vi "Load Material Dialog.vi"(8 "error in":errorcluster, 9 "Material.Details":T2={"Font Name"="Segoe UI", "Button.Font Size"=30, "Message.Font Size"=30, "Message.Justification"=enum."Center", "Picture Background"=16777216}, 10 "Material.Scheme":T1) -> (0 "error out":errorcluster, 3 "Theme Obj":refnum<class "Theme.lvclass">)   [LabVIEW 2021, in "Theme.lvclass"]
doc: "Load a theme from a material file supported by the TSC Material Library:\n\nhttps://github.com/danielcoons/tsc-material-theme\nhttps://www.vipm.io/package/tsc_lib_tsc_material_theme/\n\n<b>Code Developed By:</b>\nTechnology Service Corporation\n1983 S Liberty Drive\nBloomington, IN 47403\nPhone: 812 558-7100\nwww.tsc.com/atcs\n\nDeveloper:\nDaniel Coons"
uses:
  Theme.lvclass
  Material.Details--typedef.ctl
  Material.Scheme--typedef.ctl
  Button colors--typedef.ctl
  message box--typdef.ctl
  Dialog colors--typedef.ctl
  Theme.lvclass/Theme.ctl
  Popup/PopUp Theme Global.vi
  Popup/Popup.lvclass
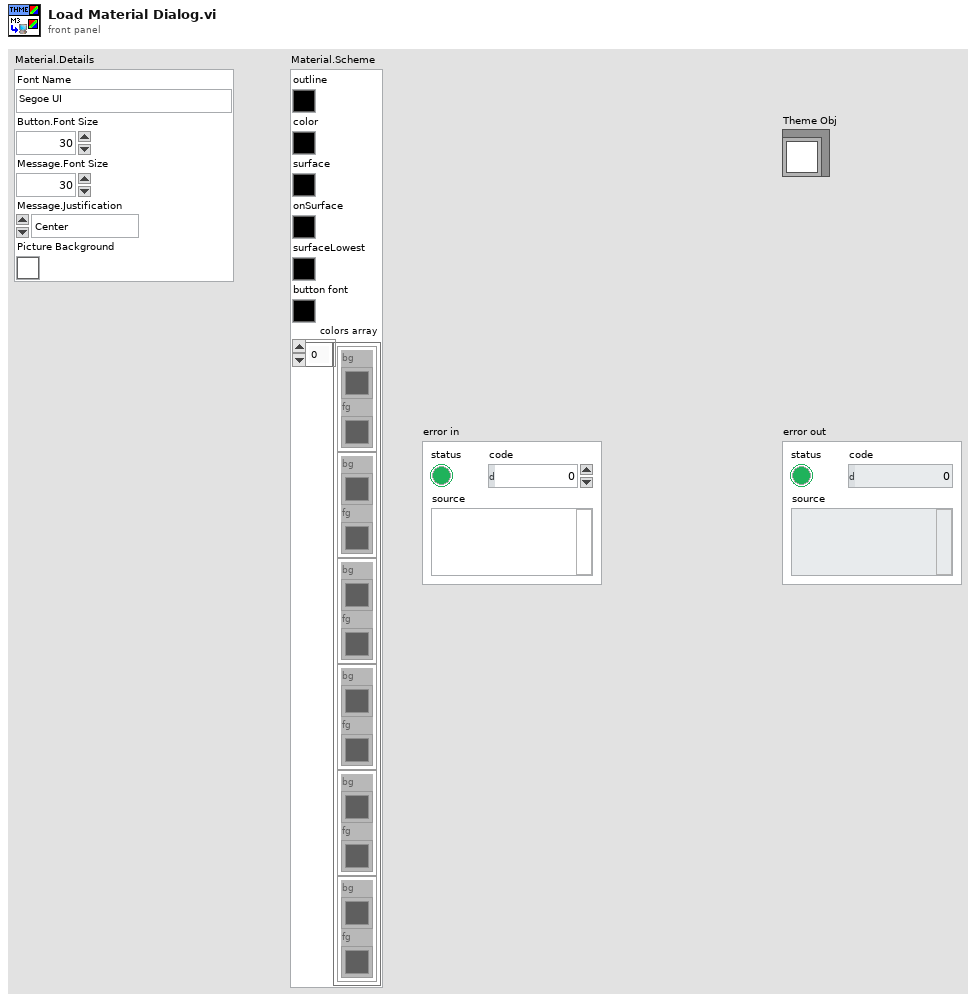
[diagram p1: front panel]
types:
  T1 = typedef "Theme.lvclass/Material.Scheme--typedef.ctl" = cluster{"outline":u32, "color":u32, "surface":u32, "onSurface":u32, "surfaceLowest":u32, "button font":u32, "colors array":cluster{"bg":u32, "fg":u32}[]}
  T2 = typedef "Theme.lvclass/Material.Details--typedef.ctl" = cluster{"Font Name":string, "Button.Font Size":u32, "Message.Font Size":u32, "Message.Justification":enum16{"Left", "Center", "Right"}, "Picture Background":u32}
  T3 = typedef "Theme.lvclass/Dialog colors--typedef.ctl" = cluster{"Header":u32, "Background":u32, "Picture Background":u32}
  T4 = typedef "Theme.lvclass/message box--typdef.ctl" = cluster{"Text.Font Name":string, "Text.Font Size":u32, "Color":u32, "Text.Justification":enum16{"Left", "Center", "Right"}, "messge color":cluster{"border":u32, "fill":u32}}
  T5 = typedef "Theme.lvclass/Button colors--typedef.ctl" = cluster{"false color":cluster{"border":u32, "fill":u32}, "hover color":cluster{"border":u32, "fill":u32}, "press color":cluster{"border":u32, "fill":u32}, "Boolean Text":u32, "Text.Font Name":string, "Text.Font Size":u32, "Bold?":bool, "Itallic?":bool}
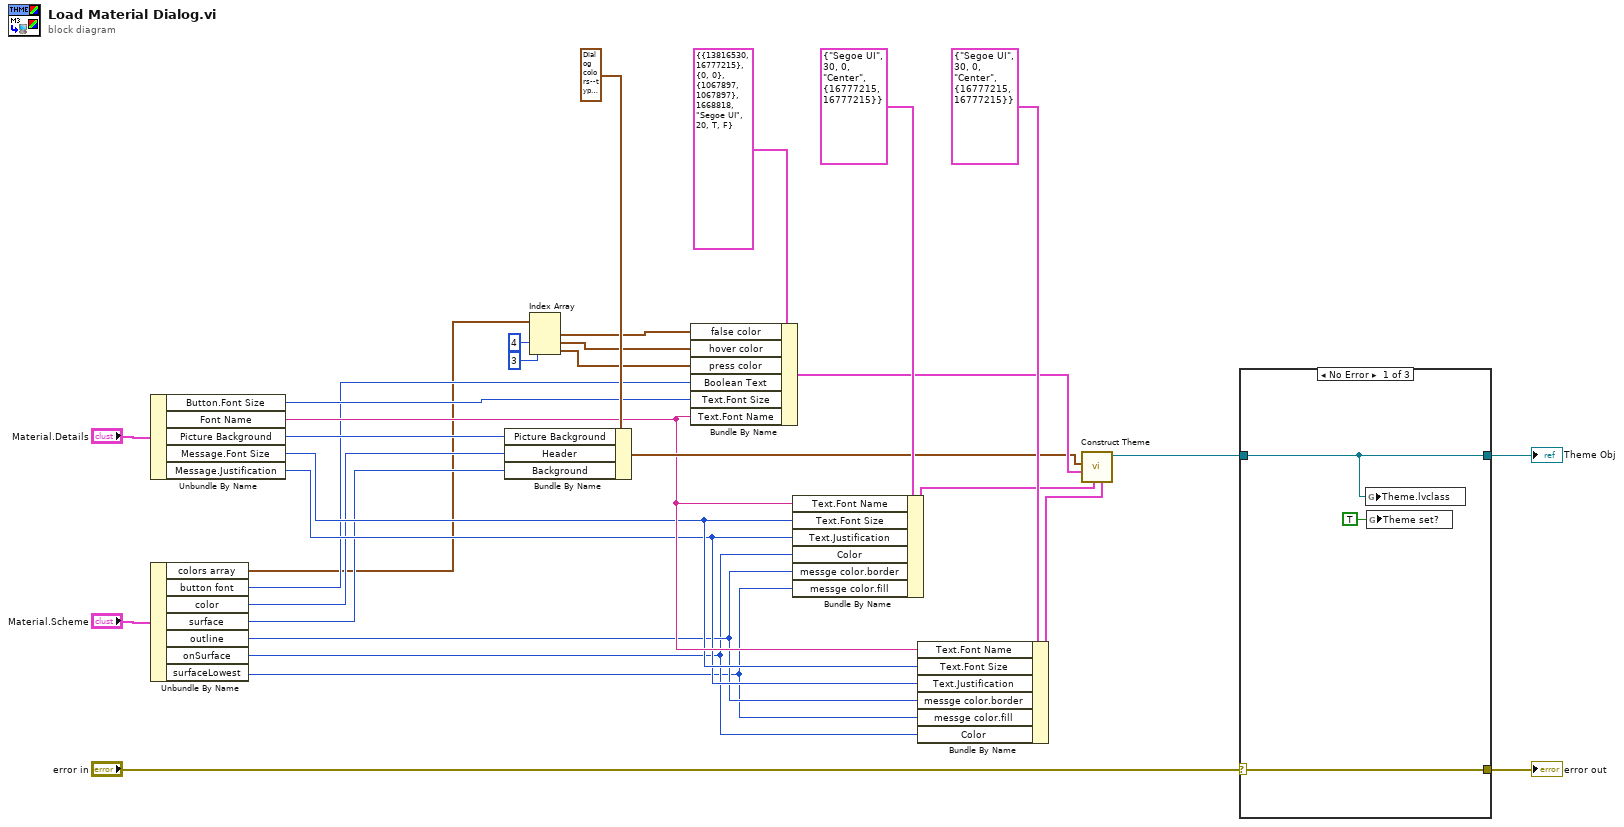
[diagram p0: block diagram]
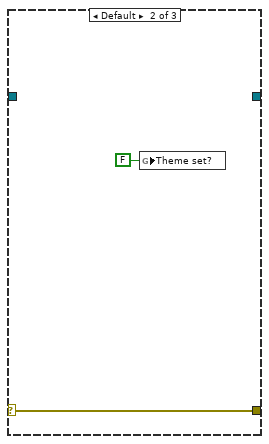
[diagram p2: hidden frame]
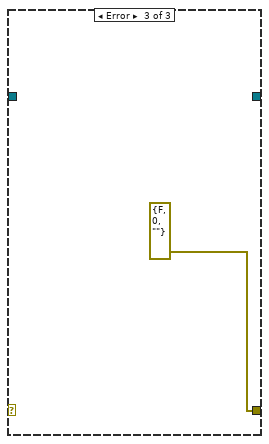
[diagram p3: hidden frame]
diagram:
  n1 = Unbundle By Name("Material.Details") -> ("Button.Font Size"=w13:u32, "Font Name"=w12:string, "Picture Background"=w11:u32, "Message.Font Size"=w10:u32, "Message.Justification"=w9:enum16{"Left", "Center", "Right"})
  n2 = Unbundle By Name("Material.Scheme") -> ("colors array"=w1:cluster{"bg":u32, "fg":u32}[], "button font"=w2:u32, "color"=w7:u32, "surface"=w5:u32, "outline"=w6:u32, "onSurface"=w4:u32, "surfaceLowest"=w3:u32)
  n3 = Bundle By Name(cluster=T3 {"Header"=1668818, "Background"=1668818, "Picture Background"=16777216} ("dialog colors"), "Picture Background"=w11, "Header"=w7, "Background"=w5) -> (w20:T3)
  n4 = Index Array(array=w1, index #2=4 ("index"), index #3=3 ("index")) -> (element #1=w19:cluster{"bg":u32, "fg":u32}, element #2=w16:cluster{"bg":u32, "fg":u32}, element #3=w15:cluster{"bg":u32, "fg":u32})  [unwired: 1 in]
  n5 = Bundle By Name(cluster=T5 {"false color"={"border"=13816530, "fill"=16777215}, "hover color"={"border"=0, "fill"=0}, "press color"={"border"=1067897, "fill"=1067897}, "Boolean Text"=1668818, "Text.Font Name"="Segoe UI", "Text.Font Size"=20, "Bold?"=TRUE, "Itallic?"=FALSE} ("button colors"), "false color"=w19, "hover color"=w16, "press color"=w15, "Boolean Text"=w2, "Text.Font Size"=w13, "Text.Font Name"=w12) -> (w22:T5)
  n6 = Bundle By Name(cluster=T4 {"Text.Font Name"="Segoe UI", "Text.Font Size"=30, "Color"=0, "Text.Justification"=enum."Center", "messge color"={"border"=16777215, "fill"=16777215}} ("message font"), "Text.Font Name"=w12, "Text.Font Size"=w10, "Text.Justification"=w9, "Color"=w4, "messge color.border"=w6, "messge color.fill"=w3) -> (w23:T4)
  n7 = Bundle By Name(cluster=T4 {"Text.Font Name"="Segoe UI", "Text.Font Size"=30, "Color"=0, "Text.Justification"=enum."Center", "messge color"={"border"=16777215, "fill"=16777215}} ("input"), "Text.Font Name"=w12, "Text.Font Size"=w10, "Text.Justification"=w9, "messge color.border"=w6, "messge color.fill"=w3, "Color"=w4) -> (w24:T4)
  n8 = call "Construct Theme.vi"("input"=w24, "message font"=w23, "button colors"=w22, "dialog colors"=w20) -> ("Theme out"=w28:refnum<class "Theme.lvclass">)  [unwired: 6 in, 1 out]
  n9 = case shown="No Error" "error in" {
    selector: "error in" -> [w34 w36 _]
    tunnel: [w34 w36 errorcluster {"status"=FALSE, "code"=0, "source"=""} ("error IO")] -> w30
    tunnel: w28 -> [w33 _ _]
    tunnel: [w33 _ _] -> w29
    frame No Error {
      n10 = global write "PopUp Theme Global.vi" "Theme.lvclass"(w33) -> ()
      n11 = global write "PopUp Theme Global.vi" "Theme set?"(TRUE ("Theme set?")) -> ()
    }
    frame Default {
      n12 = global write "PopUp Theme Global.vi" "Theme set?"(FALSE ("Theme set?")) -> ()
    }
    frame Error {
    }
  }
  "error out" <- w30
  "Theme Obj" <- w29
